vi "Periodic Tasks.vi"() -> ()   [LabVIEW 2012]
doc: "This VI runs in parallel to other tasks. It can contain as many user-defined periodic loops as you need. These can carry out PID or other sorts of timed response."
uses:
  <vilib>/Rock Robotics/SystemInterfaces/Utilities/FPGA_UtilitiesLED Source.ctl
  <vilib>/Rock Robotics/SystemInterfaces/Utilities/FPGA_UtilitiesLED State.ctl
  Autonomous_Routine_Global.vi
  <vilib>/Rock Robotics/WPI/Joystick/WPI_JoystickGetSetRefNum.vi
  Robot Global Data.vi
panel:
  in  "FireTime(ms)":dbl(slide)=1000.0 scale=0.0..1000.0
  out "Voltage":dbl(knob) scale=0.0..5.0
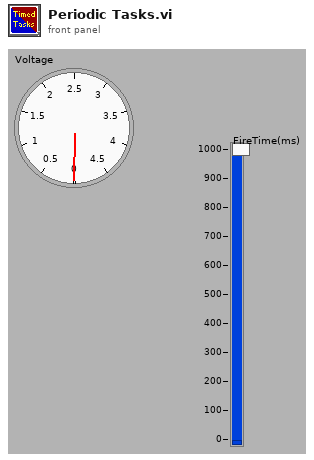
[diagram p1: front panel]
types:
  T1 = typedef "WPI_AnalogChannelDevRef.ctl" = cluster{"DevStatus":errorcluster, "Analog Module":T2, "Analog Channel":T3}
  T2 = typedef "FPGA_TypedefAnalogModule.ctl" = enum16{"Analog Module 1", "Analog Module 2"}
  T3 = typedef "FPGA_AIChannel.ctl" = enum8{"AI 1", "AI 2", "AI 3", "AI 4", "AI 5", "AI 6", "AI 7", "AI 8", "Invalid"}
  T4 = typedef "FPGA_UtilitiesLED State.ctl" = enum16{"Off", "On", "Toggle"}
  T5 = typedef "FPGA_UtilitiesLED Source.ctl" = enum16{"User LED", "FPGA LED"}
  T6 = typedef "WPI_JoystickDevRef.ctl" = cluster{"Device":T7}
  T7 = typedef "WPI_JoystickDeviceEnum.ctl" = enum16{"USB 1", "USB 2", "USB 3", "USB 4", "Kinect 1", "Kinect 2"}
  T8 = typedef "WPI_JoystickButtonState.ctl" = cluster{"Button 1":bool, "Button 2":bool, "Button 3":bool, "Button 4":bool, "Button 5":bool, "Button 6":bool, "Button 7":bool, "Button 8":bool, "Button 9":bool, "Button 10":bool, "Button 11":bool, "Button 12":bool}
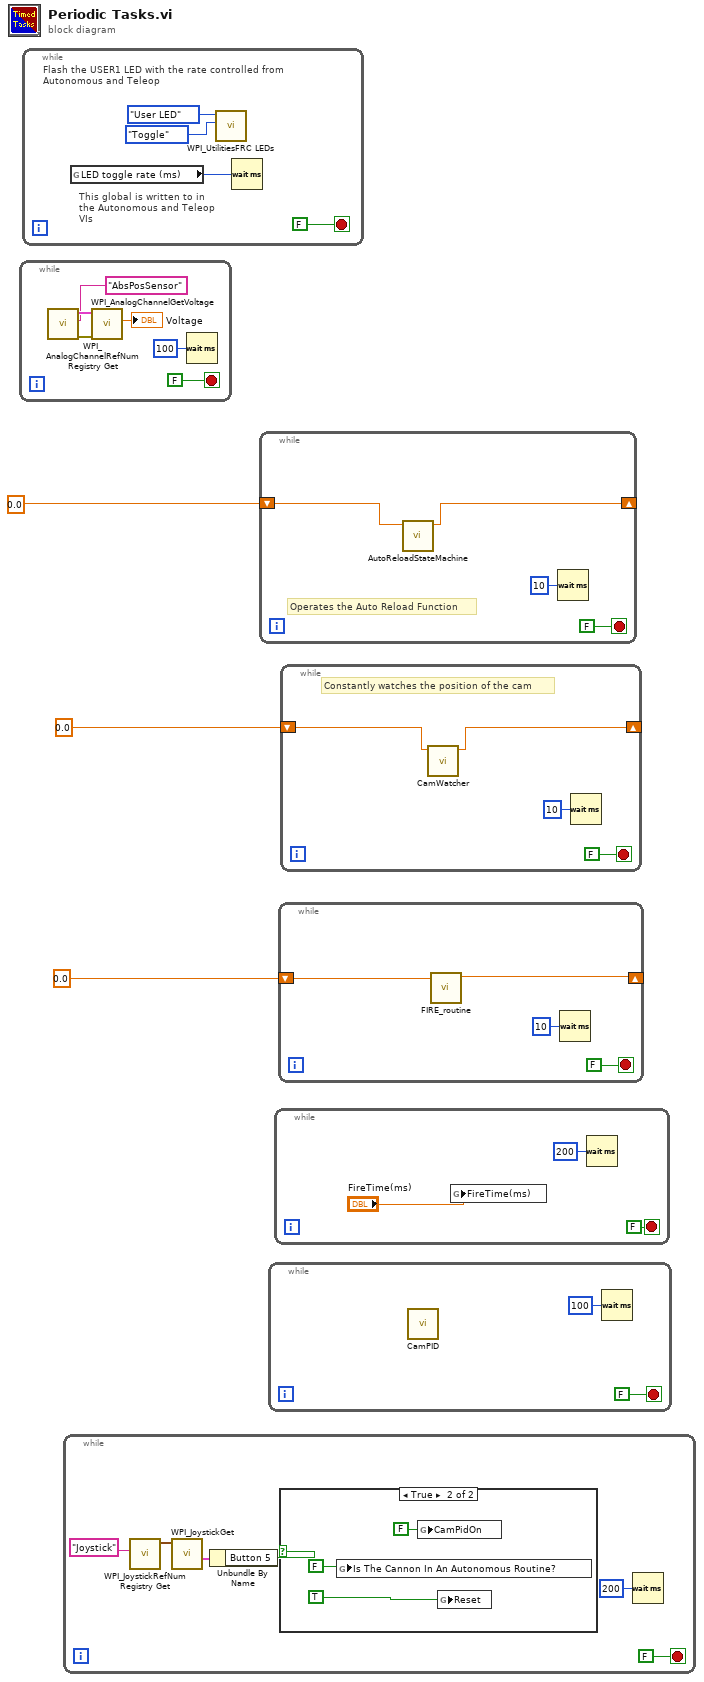
[diagram p0: block diagram]
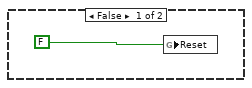
[diagram p2: hidden frame]
diagram:
  n1 = while {
    stop <- FALSE stop-if-true
    n2 = call <vilib>:"WPI_AnalogChannelRefNum Registry Get.vi"("refnum name"="AbsPosSensor") -> ("error out"=w7:errorcluster, "AIDeviceRef"=w6:T1)  [unwired: 9 in]
    n3 = call <vilib>:"WPI_AnalogChannelGetVoltage.vi"("error in (no error)"=w7, "AIDeviceRef"=w6) -> ("Voltage"=→"Voltage":dbl)  [unwired: 7 in, 2 out]
    n4 = Wait (ms)(milliseconds to wait=u32 100) -> ()  [unwired: 1 out]
  }
  n5 = while {
    stop <- FALSE stop-if-true
    # "This global is written to in the Autonomous and Teleop VIs"
    # "Flash the USER1 LED with the rate controlled from Autonomous and Teleop"
    n6 = global read "Robot Global Data.vi" "LED toggle rate (ms)"() -> (w10:u32)
    n7 = call <vilib>:"WPI_UtilitiesFRC LEDs.vi"("State"=FPGA_UtilitiesLED_State."Toggle", "LED Type"=FPGA_UtilitiesLED_Source."User LED") -> ()  [unwired: 1 in, 9 out]
    n8 = Wait (ms)(milliseconds to wait=w10) -> ()  [unwired: 1 out]
  }
  n9 = while {
    stop <- FALSE stop-if-true
    n10 = call <vilib>:"WPI_JoystickRefNum Registry Get.vi"("refnum name"="Joystick") -> ("JoystickDevRef"=w17:T6)  [unwired: 9 in, 1 out]
    n11 = call <vilib>:"WPI_JoystickGet.vi"("JoystickDevRef"=w17) -> ("Buttons"=w16:T8)  [unwired: 4 in, 2 out]
    n12 = Unbundle By Name(w16) -> ("Button 5"=w15:bool)
    n13 = case shown="True" w15 {
      frame False {
        n14 = global write "Autonomous_Routine_Global.vi" "Reset"(FALSE ("CamPidOn")) -> ()
      }
      frame True {
        n15 = global write "Autonomous_Routine_Global.vi" "Is The Cannon In An Autonomous Routine?"(FALSE ("CamPidOn")) -> ()
        n16 = global write "Autonomous_Routine_Global.vi" "CamPidOn"(FALSE ("CamPidOn")) -> ()
        n17 = global write "Autonomous_Routine_Global.vi" "Reset"(TRUE ("CamPidOn")) -> ()
      }
    }
    n18 = Wait (ms)(milliseconds to wait=u32 200) -> ()  [unwired: 1 out]
  }
  n19 = while {
    shift-right: [w25] -> _
    shift-left: 0.0 -> [w26]
    stop <- FALSE stop-if-true
    # "Operates the Auto Reload Function"
    n20 = call "AutoReloadStateMachine.vi"("Current State In"=w26) -> ("Current State Out"=w25:dbl)  [unwired: 10 in]
    n21 = Wait (ms)(milliseconds to wait=u32 10) -> ()  [unwired: 1 out]
  }
  n22 = while {
    stop <- FALSE stop-if-true
    n23 = call "CamPID.vi"() -> ()  [unwired: 12 in]
    n24 = Wait (ms)(milliseconds to wait=u32 100) -> ()  [unwired: 1 out]
  }
  n25 = while {
    stop <- FALSE ("stop") stop-if-true
    n26 = global write "Autonomous_Routine_Global.vi" "FireTime(ms)"("FireTime(ms)") -> ()
    n27 = Wait (ms)(milliseconds to wait=u32 200) -> ()  [unwired: 1 out]
  }
  n28 = while {
    shift-right: [w35] -> _
    shift-left: 0.0 ("StateOut") -> [w36]
    stop <- FALSE stop-if-true
    n29 = call "FIRE_routine.vi"("StateIn"=w36) -> ("StateOut"=w35:dbl)  [unwired: 10 in]
    n30 = Wait (ms)(milliseconds to wait=u32 10) -> ()  [unwired: 1 out]
  }
  n31 = while {
    shift-right: [w37] -> _
    shift-left: 0.0 ("Rotation Count") -> [w38]
    stop <- FALSE stop-if-true
    # "Constantly watches the position of the cam"
    n32 = call "CamWatcher.vi"("Rotation Count"=w38) -> ("Rotation Count"=w37:dbl)  [unwired: 10 in]
    n33 = Wait (ms)(milliseconds to wait=u32 10) -> ()  [unwired: 1 out]
  }
